vi "ROI entry- extract anc check ROI data.vi"(8 "error in (no error)":errorcluster, 10 "ROI File data":dbl[][](array[numeric]), 11 "Old ROI file path":path) -> (0 "error out":errorcluster, 1 "Latest AOL Z values":dbl[](array[numeric]), 2 "Last ROI Enum":T1, 3 "Array":T2[](array[typedef]) {"FOV" min=1.0 max=10.0 step=1.0; "Frame Size" min=1.0 max=10.0 step=1.0; "Laser Power" min=1.0 max=10.0 step=0.10000000149011612; "Rel. Resolution" min=1.0 max=10.0 step=1.0; "POI Dwell time" min=1.0 max=10.0 step=0.10000000149011612; "Zoom" min=1.0 max=10.0 step=0.10000000149011612}, 5 "ROI type consistent":bool)   [LabVIEW 2020]
uses:
  Typedefs/ROI spec.ctl
  Typedefs/ROI ID Enum.ctl
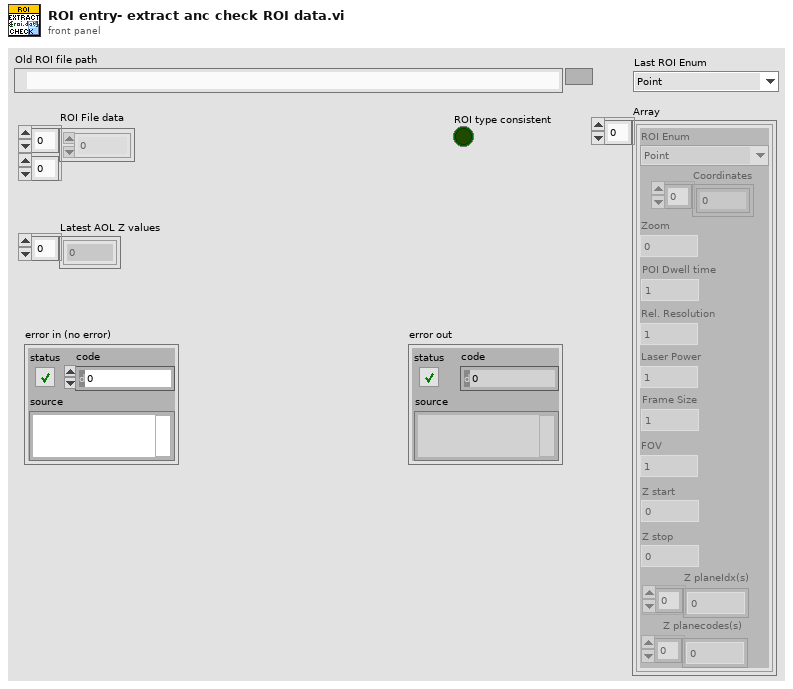
[diagram p1: front panel]
types:
  T1 = typedef "ROI ID Enum.ctl" = enum16{"Point", "MiniScan", "Comp. MiniScan", "Rectangle", "Comp. volume", "Arb. plane point", "None"}
  T2 = typedef "ROI spec.ctl" = cluster{"ROI Enum":T1, "Coordinates":i32[], "Zoom":dbl, "POI Dwell time":dbl, "Rel. Resolution":dbl, "Laser Power":dbl, "Frame Size":dbl, "FOV":dbl, "Z start":dbl, "Z stop":dbl, "Z planeIdx(s)":i32[], "Z planecodes(s)":u8[]}
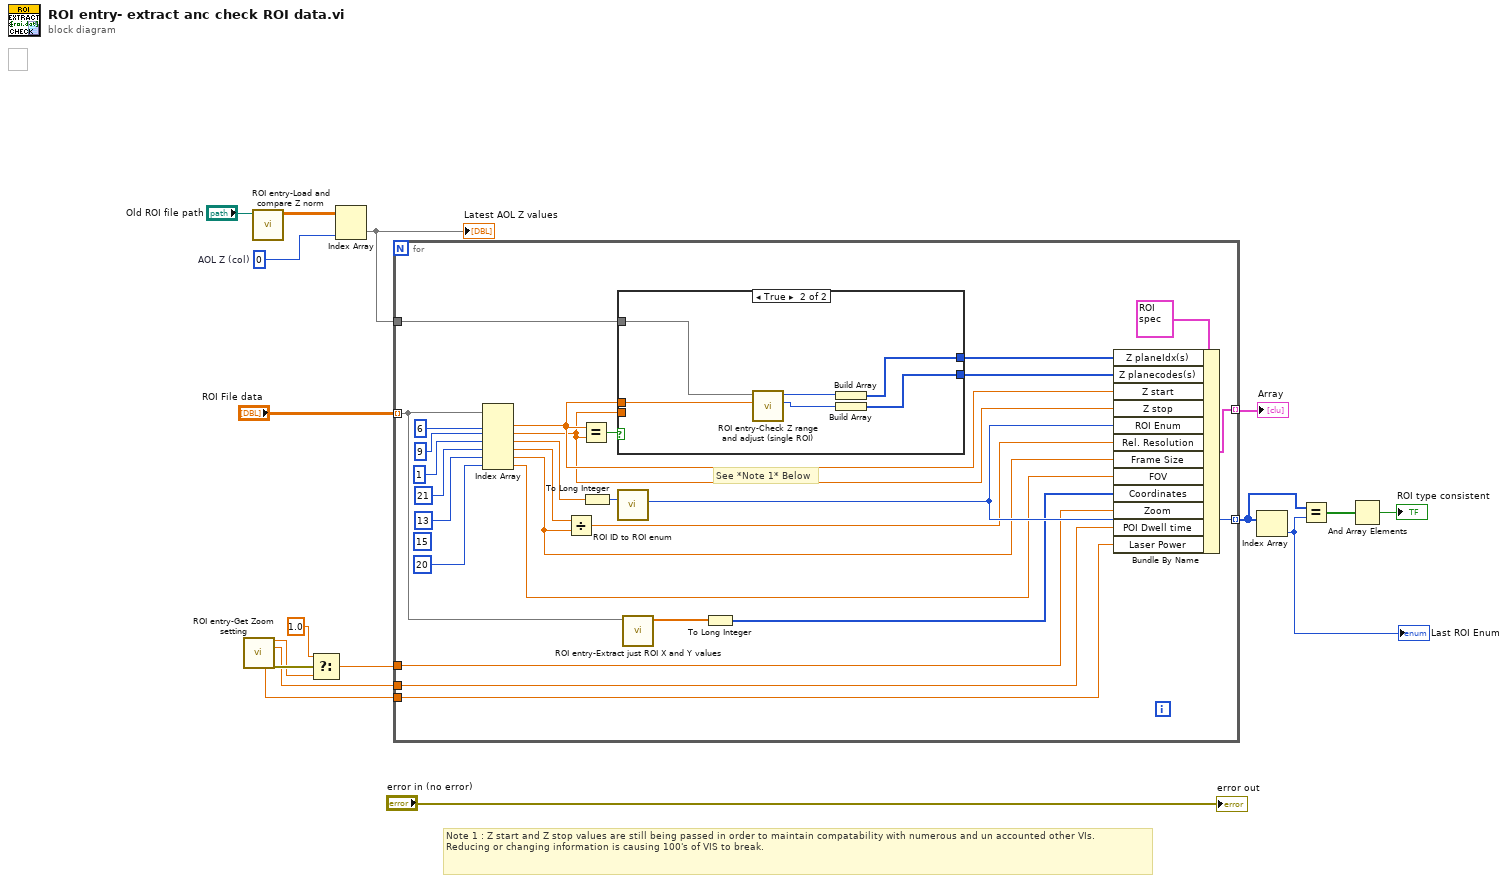
[diagram p0: block diagram]
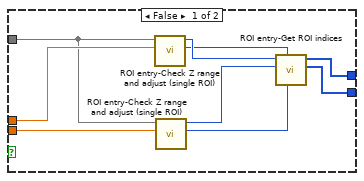
[diagram p2: hidden frame]
diagram:
  w15 = 0  # AOL Z (col)
  # "Note 1 : Z start and Z stop values are still being passed in order to maintain compatability with numerous and un accounted other VIs. \nReducing or changing information is causing 100's of VIS to break."
  n1 = call "ROI entry-Get Zoom setting.vi"() -> ("Zoom Value"=w3:dbl, "POI dwell time"=w2:dbl, "Laser Power"=w1:dbl, "error out"=w13:errorcluster)  [unwired: 7 in, 5 out]
  n2 = call "ROI entry-Load and compare Z norm.vi"("Old ROI file path"="Old ROI file path") -> ("Latest Zplane_Pockels_Values file data (header removed)"=w16:dbl[][])  [unwired: 4 in, 6 out]
  n3 = Select(t=1.0, s=w13, f=w3) -> (s? t:f=w11:dbl)
  n4 = Index Array(array=w16, index (col)=w15) -> (element=w9:dbl[])  [unwired: 1 in]
  "Latest AOL Z values" <- w9
  n5 = for {
    tunnel: "ROI File data" -> [w39] mode=indexing
    tunnel: w11 -> [w28]
    tunnel: [w36] -> w10 mode=indexing
    tunnel: w9 -> [w35]
    tunnel: [w32] -> w8 mode=indexing
    tunnel: w2 -> [w22]
    tunnel: w1 -> [w18]
    (unwired) 15 ("index")
    # "See *Note 1* Below"
    n6 = Index Array(array=w39, index #1=6, index #2=9, index #3=1 ("index"), index #4=21 ("index"), index #5=13 ("index"), index #6=20 ("index")) -> (element #1=w30:dbl, element #2=w29:dbl, element #3=w37:dbl, element #4=w24:dbl, element #5=w21:dbl, element #6=w19:dbl)
    n7 = Divide(x=w24, y=w21) -> (x/y=w23:dbl)
    n8 = Equal?(x=w30, y=w29) -> (x = y?=w41:bool)
    n9 = To Long Integer(number=w37) -> (32bit integer=w38:i32)
    n10 = case shown="True" w41 {
      tunnel: w30 -> [w53 w58]
      tunnel: w29 -> [w51 _]
      tunnel: w35 -> [w52 w59]
      tunnel: [w46 w56] -> w34
      tunnel: [w45 w54] -> w33
      frame False {
        n11 = call "ROI entry-Check Z range and adjust (single ROI).vi"("AOL Z plane value"=w53, "Latest Zplane_Pockels_Values file data (header removed)"=w52) -> ("Z plane code"=w49:u8, "Z plane Index"=w50:i32)  [unwired: 7 in, 1 out]
        n12 = call "ROI entry-Check Z range and adjust (single ROI).vi"("AOL Z plane value"=w51, "Latest Zplane_Pockels_Values file data (header removed)"=w52) -> ("Z plane code"=w47:u8, "Z plane Index"=w48:i32)  [unwired: 7 in, 1 out]
        n13 = call "ROI entry-Get ROI indices.vi"("Z stop code"=w47, "Z start code"=w49, "Z stop index"=w48, "Z start Index"=w50) -> ("Z codes"=w45:u8[], "Z Idx(s)"=w46:i32[])  [unwired: 6 in]
      }
      frame True {
        n14 = call "ROI entry-Check Z range and adjust (single ROI).vi"("AOL Z plane value"=w58, "Latest Zplane_Pockels_Values file data (header removed)"=w59) -> ("Z plane code"=w55:u8, "Z plane Index"=w57:i32)  [unwired: 7 in, 1 out]
        n15 = Build Array(w57) -> (w56:i32[])
        n16 = Build Array(w55) -> (w54:u8[])
      }
    }
    n17 = call "ROI ID to ROI enum.vi"("ROI ID"=w38) -> ("ROI Enum"=w32:T1)  [unwired: 6 in]
    n18 = call "ROI entry-Extract just ROI X and Y values.vi"("Single ROI component data"=w39) -> ("X and Y values array"=w31:dbl[])  [unwired: 10 in]
    n19 = To Long Integer(number=w31) -> (32bit integer=w27:i32[])
    n20 = Bundle By Name(cluster=T2 {"ROI Enum"=enum."Point", "Coordinates"=[], "Zoom"=1.0, "POI Dwell time"=1.0, "Rel. Resolution"=1.0, "Laser Power"=1.0, "Frame Size"=1.0, "FOV"=1.0, "Z start"=0.0, "Z stop"=0.0, "Z planeIdx(s)"=[], "Z planecodes(s)"=[]} ("input cluster"), "Z planeIdx(s)"=w34, "Z planecodes(s)"=w33, "Z start"=w30, "Z stop"=w29, "ROI Enum"=w32, "Rel. Resolution"=w23, "Frame Size"=w21, "FOV"=w19, "Coordinates"=w27, "Zoom"=w28, "POI Dwell time"=w22, "Laser Power"=w18) -> (w36:T2)
  }
  "Array" <- w10
  n21 = Index Array(array=w8) -> (element=w5:T1)  [unwired: 1 in]
  "Last ROI Enum" <- w5
  n22 = Equal?(x=w8, y=w5) -> (x = y?=w7:bool[])
  n23 = And Array Elements(Boolean array=w7) -> (logical AND=→"ROI type consistent":bool)
  "error out" <- "error in (no error)"
